vi "3.2.1.8-VectorNav GenCom.vi"(0 "State":enum16{"Send", "Receive"}(ring), 1 "Local Clock: Clk":i8, 2 "Foreign Clock: Clk*":i8, 3 "Out of Message":bool, 4 "This is the Last Byte to Read":bool) -> (5 "Send New Data":bool, 6 "New Local Clock: Clk":i8, 7 "Store New Data":bool)   [LabVIEW 2010]
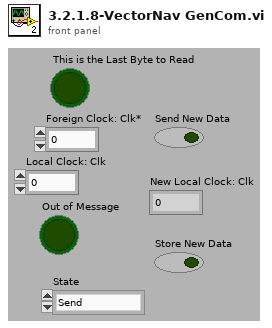
[diagram p1: front panel]
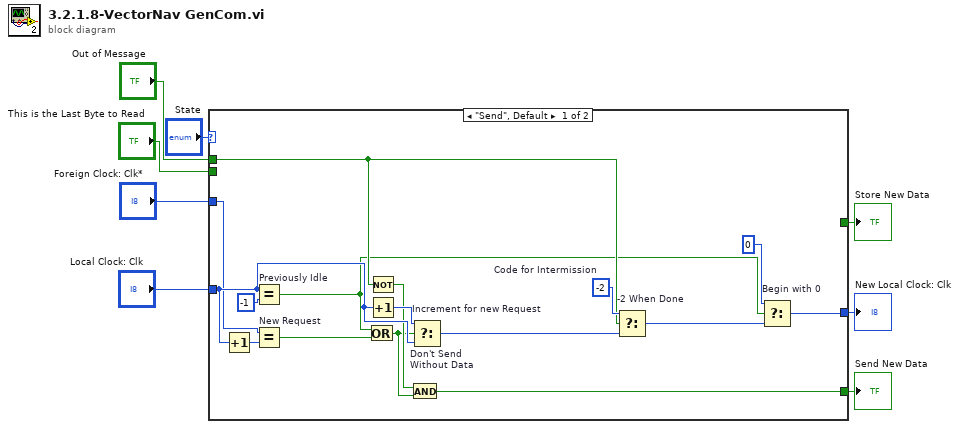
[diagram p0: block diagram]
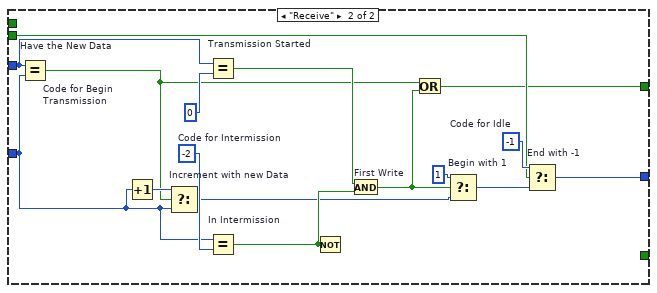
[diagram p2: hidden frame]
diagram:
  n1 = case shown="\"Send\", Default" "State" {
    tunnel: [_ w32] -> w8
    tunnel: "Foreign Clock: Clk*" -> [w20 w33]
    tunnel: [w12 w34] -> w5
    tunnel: "Local Clock: Clk" -> [w22 w31]
    tunnel: "This is the Last Byte to Read" -> [_ w39]
    tunnel: "Out of Message" -> [w13 _]
    tunnel: [w15 _] -> w1
    frame "Send", Default {
      w19 = i8 -2  # Code for Intermission
      n2 = Increment(x=w22) -> (x+1=w21:i8)
      n3 = Equal? "Previously Idle"(x=w22, y=i8 -1) -> (x = y?=w9:bool)
      n4 = Equal? "New Request"(x=w20, y=w21) -> (x = y?=w16:bool)
      n5 = Or(x=w9, y=w16) -> (x .or. y?=w10:bool)
      n6 = Not(x=w13) -> (.not. x?=w14:bool)
      n7 = Increment(x=w22) -> (x+1=w23:i8)
      n8 = And "Don't Send\nWithout Data"(x=w14, y=w10) -> (x .and. y?=w15:bool)
      n9 = Select "Increment for new Request"(t=w23, s=w10, f=w22) -> (s? t:f=w18:i8)
      n10 = Select "-2 When Done"(t=w19, s=w13, f=w18) -> (s? t:f=w17:i8)
      n11 = Select "Begin with 0"(t=i8 0, s=w9, f=w17) -> (s? t:f=w12:i8)
    }
    frame "Receive" {
      w37 = i8 0  # Code for Begin Transmission
      w38 = i8 -2  # Code for Intermission
      w40 = i8 -1  # Code for Idle
      n12 = Equal? "Have the New Data"(x=w33, y=w31) -> (x = y?=w29:bool)
      n13 = Increment(x=w31) -> (x+1=w30:i8)
      n14 = Select "Increment with new Data"(t=w30, s=w29, f=w31) -> (s? t:f=w28:i8)
      n15 = Equal? "Transmission Started"(x=w33, y=w37) -> (x = y?=w36:bool)
      n16 = Equal? "In Intermission"(x=w31, y=w38) -> (x = y?=w35:bool)
      n17 = Not(x=w35) -> ()  [unwired: 1 out]
      n18 = And "First Write"(x=w36, y=w35) -> (x .and. y?=w26:bool)
      n19 = Or(x=w29, y=w26) -> (x .or. y?=w32:bool)
      n20 = Select "Begin with 1"(t=i8 1, s=w26, f=w28) -> (s? t:f=w25:i8)
      n21 = Select "End with -1"(t=w40, s=w39, f=w25) -> (s? t:f=w34:i8)
    }
  }
  "Send New Data" <- w1
  "Store New Data" <- w8
  "New Local Clock: Clk" <- w5
